vi "mks946_get_pressure.vi"(6 "err_in":errorcluster, 7 "mks946_visa":refnum<visa-resource-name>="COM3", 10 "mks946_ch":dbl=1.0, 11 "mks946_id":i32=253) -> (0 "mks946_st":bool=TRUE, 3 "mks946_res":T1={"res_ch"=enum."ERR", "res_val"=0.0, "res_id"=0, "res_msg"="N/A"}, 4 "err_out":errorcluster={"status"=FALSE, "code"=1073676294, "source"="VISA Read in thcd_get_chan.vi"}, 5 "mks946_visa":refnum<visa-resource-name>="COM3")   [LabVIEW 2020]
uses:
  mks946_controls/ctrl_mks946_res.ctl
panel:
  in  "mks946_comm":string="PR"
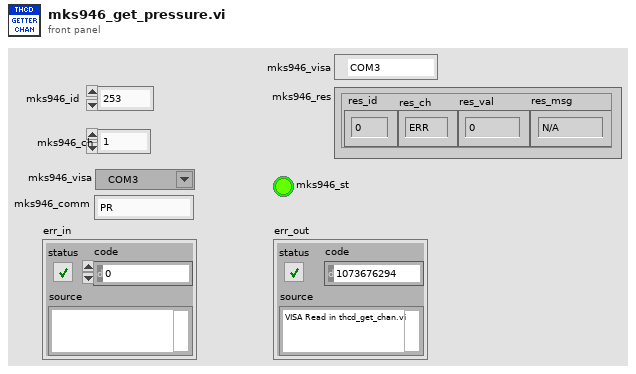
[diagram p1: front panel]
types:
  T1 = typedef "ctrl_mks946_res.ctl" = cluster{"res_ch":enum8{"ERR", "1", "2", "3", "4", "5", "6"}, "res_val":dbl, "res_id":u8, "res_msg":string}
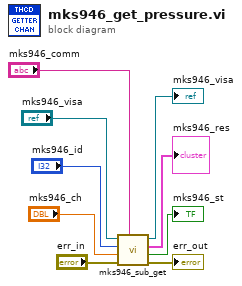
[diagram p0: block diagram]
diagram:
  n1 = call "mks946_sub_get.vi"("mks946_comm"="mks946_comm", "error in (no error)"="err_in", "mks946_ch"="mks946_ch", "mks946_id"="mks946_id", "VISA_ref_in"="mks946_visa") -> ("error out"=→"err_out":errorcluster, "Boolean"=→"mks946_st":bool, "mks946_res_def"=→"mks946_res":T1, "VISA_ref_out"=→"mks946_visa":refnum<visa-resource-name>)  [unwired: 3 in]
